vi "Write_Env.vi"(0 "COM Bluegiga in":refnum<visa-resource-name>, 1 "Handle table":string[][](array[string]), 3 "Service UUID":string, 4 "Characteristic UUID":string, 5 "Registro Completo":u8[](array[numeric]), 7 "error in (no error)":errorcluster, 8 "Intervalo Temperatura":u16, 9 "Intensidad Verde":u8, 10 "Intervalo Humedad":u16, 11 "Intensidad Azul":u8, 12 "Intervalo Presion":u16, 14 "Intervalo Color":u16, 15 "Connection Status":T1={"MAC Address"="", "cnx handle"=0, "cnx flags"=0, "Address Type"=125, "Connection Interval (ms)"=125, "Timeout(ms)"=125, "Latency"=0, "bonding handle"=0} {"Address Type" items=["Public", "Random"]}, 16 "Modo Aire":u8, 18 "Intensidad Rojo":u8) -> (20 "COM Bluegiga out":refnum<visa-resource-name>, 27 "error out":errorcluster)   [LabVIEW 2020]
uses:
  <vilib>/BLE/type_def/connection_status_bundle.ctl
  <vilib>/BLE/type_def/address_type.ctl
  <vilib>/BLE/ble_functions/ble_write_by_service_characteristic_uint8array.vi
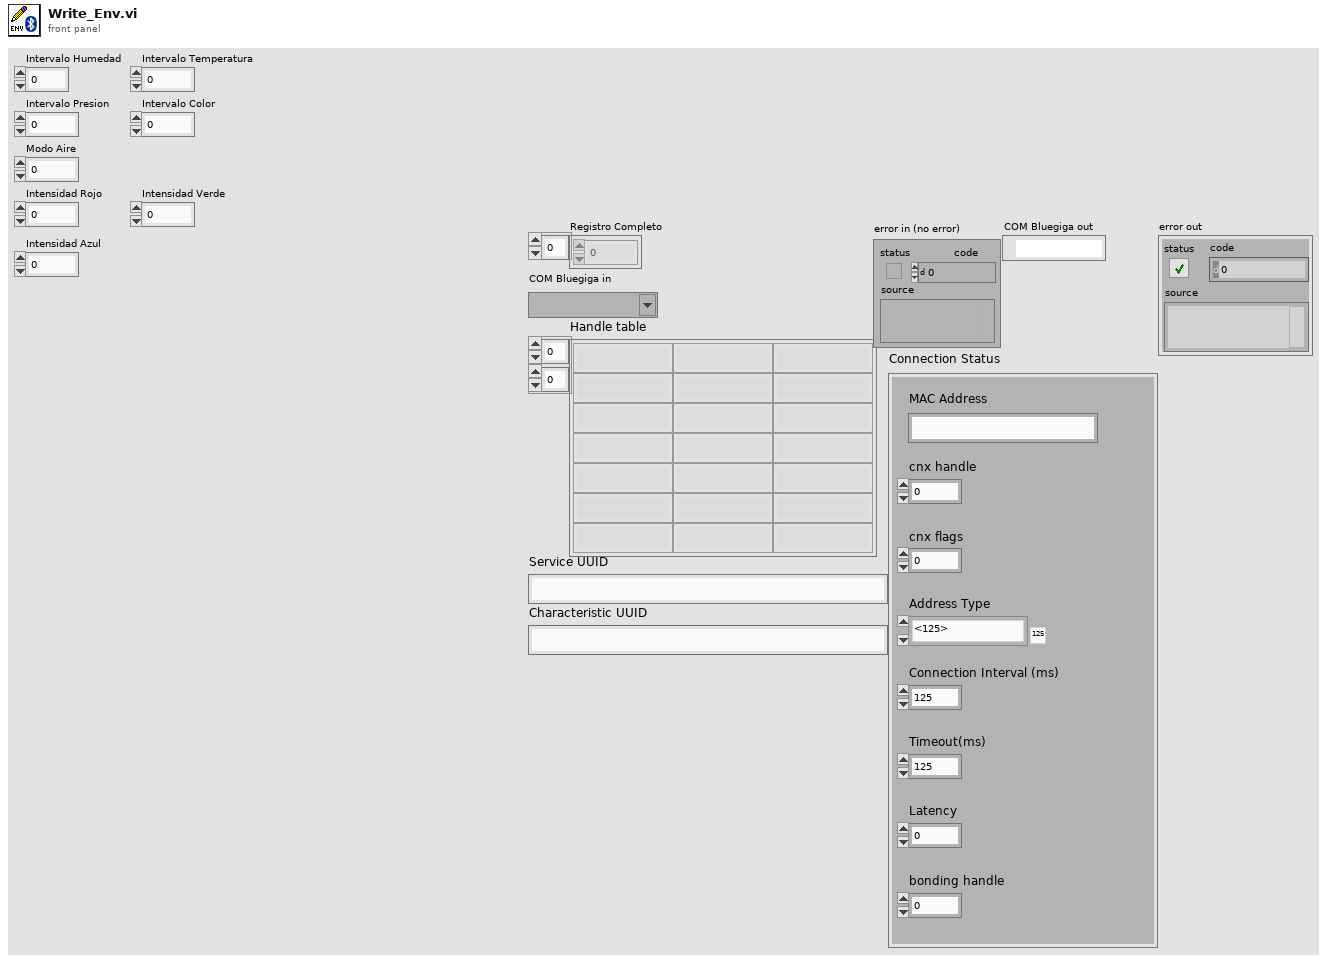
[diagram p1: front panel]
types:
  T1 = typedef "connection_status_bundle.ctl" = cluster{"MAC Address":string, "cnx handle":u8, "cnx flags":u8, "Address Type":T2, "Connection Interval (ms)":u16, "Timeout(ms)":u16, "Latency":u16, "bonding handle":u8}
  T2 = typedef "address_type.ctl" = u8
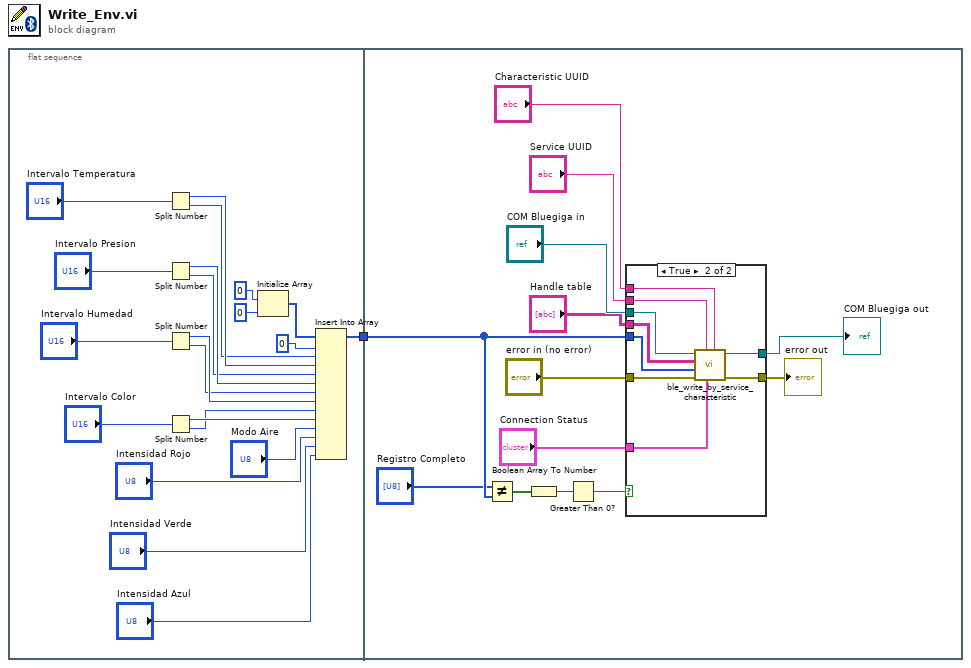
[diagram p0: block diagram]
diagram:
  n1 = flat-sequence {
    tunnel: [w22] -> w1
    tunnel: w1 -> [w24]
    frame #0 {
      n2 = Split Number(x="Intervalo Temperatura") -> (hi(x)=w15:u8, lo(x)=w14:u8)
      n3 = Split Number(x="Intervalo Presion") -> (hi(x)=w17:u8, lo(x)=w16:u8)
      n4 = Split Number(x="Intervalo Humedad") -> (hi(x)=w19:u8, lo(x)=w18:u8)
      n5 = Split Number(x="Intervalo Color") -> (hi(x)=w21:u8, lo(x)=w20:u8)
      n6 = Initialize Array(u8 0 ("element"), 0 ("dimension size")) -> (w6:u8[])
      n7 = Insert Into Array(array=w6, index=0, new element #1=w14, new element #2=w15, new element #3=w16, new element #4=w17, new element #5=w18, new element #6=w19, new element #7=w20, new element #8=w21, new element #9="Modo Aire", new element #10="Intensidad Rojo", new element #11="Intensidad Verde", new element #12="Intensidad Azul") -> (w22:u8[])
    }
    frame #1 {
      n8 = Not Equal?(x="Registro Completo", y=w24) -> (x != y?=w34:bool[])
      n9 = Boolean Array To Number(Boolean array=w34) -> (number=w35:u32)
      n10 = Greater Than 0?(x=w35) -> (x > 0?=w33:bool)
      n11 = case shown="True" w33 {
        tunnel: [w36 w46] -> w28
        tunnel: [w37 w45] -> w29
        tunnel: w24 -> [_ w44]
        tunnel: "COM Bluegiga in" -> [w37 w43]
        tunnel: "Handle table" -> [_ w42]
        tunnel: "error in (no error)" -> [w36 w41]
        tunnel: "Connection Status" -> [_ w40]
        tunnel: "Service UUID" -> [_ w39]
        tunnel: "Characteristic UUID" -> [_ w38]
        frame False {
        }
        frame True {
          n12 = call-poly <vilib>:"ble_write_by_service_characteristic.vi"("Characteristic UUID"=w38, "Connection Status"=w40, "Service UUID"=w39, "error in (no error)"=w41, "data"=w44, "Handle table"=w42, "COM Bluegiga in"=w43) -> ("error out"=w46:errorcluster, "COM Bluegiga out"=w45:refnum<visa-resource-name>)  [unwired: 3 in]
        }
      }
      "COM Bluegiga out" <- w29
      "error out" <- w28
    }
  }
